vi "Loop.Timer.vi"(11 "Loop Timer (uSec)":u32) -> (3 "Actual Loop Period (usec)":u32)   [LabVIEW 2015, in "FPGA Wizard Templates.lvlib"]
uses:
  FPGA Wizard Templates.lvlib
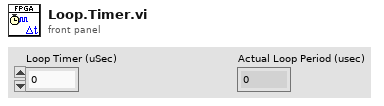
[diagram p1: front panel]
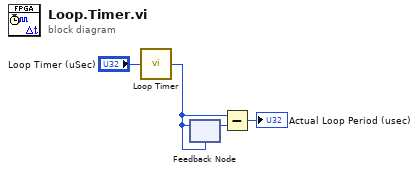
[diagram p0: block diagram]
diagram:
  n1 = call "Loop Timer"("Count(uSec)"="Loop Timer (uSec)") -> ("Tick Count(uSec)"=w3:u32)
  n2 = feedback #1(w3) -> (w2:u32)
  n3 = feedback-in #1(w3) -> ()
  n4 = Subtract(x=w3, y=w2) -> (x-y=→"Actual Loop Period (usec)":u32)
